vi "Test Method Execution Time recorded.vi"(8 "error in (no error)":errorcluster, 11 "Test Case In":refnum<class "Test Case Test.lvclass">) -> (0 "error out":errorcluster, 3 "Test Case Out":refnum<class "Test Case Test.lvclass">)   [LabVIEW 2020, in "Test Case Test.lvclass"]
uses:
  Test Case Test.lvclass
  C:/Program Files (x86)/National Instruments/LabVIEW 2020/vi.lib/Astemes/LUnit/Test Case.lvclass
  Test Doubles/Test Case Test Double/Methods.ctl
  source/Core/Result/Type.ctl
  <vilib>/Astemes/LUnit/Test Case.lvclass/Test Case.ctl
  <vilib>/Astemes/LUnit/Palette/Fail.vi
  <vilib>/Astemes/LUnit/Palette/Pass.vi
  <vilib>/Astemes/LUnit/Set Assertion Type.vi
  <vilib>/Astemes/LUnit/Add test result.vi
  <vilib>/Astemes/LUnit/LUnit Record Assertion Result.vi
  <vilib>/Astemes/LUnit/LUnit Aggregate Assertion Results.vi
  <vilib>/Astemes/LUnit/Method Result/LUnit Merge Status.vi
  <vilib>/Astemes/LUnit/LUnit Concatenate result strings.vi
  source/API/LUnit Test Case/LUnit Test Case.lvclass
  Test Doubles/Test Case Test Double/Test Case Test Double.lvclass
  <vilib>/Astemes/LUnit/Test Case.lvclass
  source/Core/Result/Result.lvlib
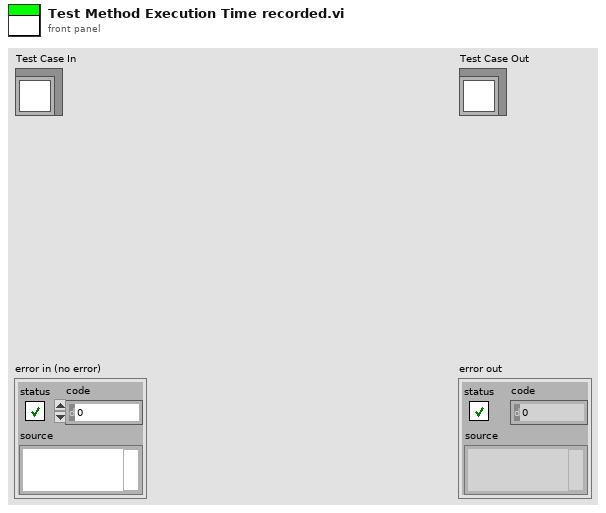
[diagram p1: front panel]
types:
  T1 = typedef "Test Case Test Double.lvclass/Methods.ctl" = enum16{"Test Failing Test.vi", "Test Passing Test.vi", "Test Error Test.vi", "Test Skip Test.vi", "Test Passing Pass If Test.vi", "Test Failing Pass If Test.vi", "Test Failing Fail If Test.vi", "Test Passing Fail If Test.vi", "Test Passing Pass If Error Test.vi", "Test Failing Pass If Error Test.vi", "Test Passing Fail If Error Test.vi", "Test Failing Fail If Error Test.vi", "Test Passing Pass If Equal Test.vi", "Test Failing Pass If Equal Test.vi", "Test Failing Fail If Equal Test.vi", "Test Passing Fail If Equal Test.vi", "Freezing Test.vi"}
  T2 = typedef "Result.lvlib/Result.ctl" = cluster{"Name":string, "Message":string, "Description":string, "Status":T3, "Result Type":T4, "Execution Time":dbl}
  T3 = typedef "Result.lvlib/Status.ctl" = enum16{"", "Passed", "Failed", "Error", "Skipped", "Setup Error", "Broken", "Teardown Error"}
  T4 = typedef "Result.lvlib/Type.ctl" = enum16{"Method", "Case", "Suite", "Pass", "Fail", "Skip", "Pass if", "Fail if", "Pass if Error", "Fail if Error", "Pass if Equal", "Fail if Equal"}
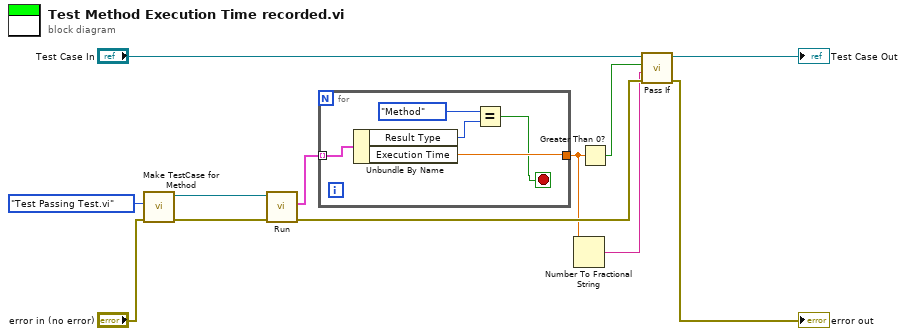
[diagram p0: block diagram]
diagram:
  n1 = call "Make TestCase for Method.vi"("error in (no error)"="error in (no error)", "Test Method"=Methods."Test Passing Test.vi") -> ("error out"=w8:errorcluster, "LUnit Test Case V2 out"=w9:refnum<class "LUnit Test Case.lvclass">)  [unwired: 8 in]
  n2 = call-dynamic "Run.vi"("error in (no error)"=w8, "LUnit Test Case In"=w9) -> ("error out"=w6:errorcluster, "Results"=w5:T2[])  [unwired: 6 in, 2 out]
  n3 = for {
    tunnel: w5 -> [w17] mode=indexing
    tunnel: [w16] -> w2
    stop <- w13 stop-if-true
    n4 = Unbundle By Name(w17) -> ("Result Type"=w14:T4, "Execution Time"=w16:dbl)
    n5 = Equal?(x=Type."Method" ("Result Type"), y=w14) -> (x = y?=w13:bool)
  }
  n6 = Number To Fractional String(number=w2) -> (F-format string=w1:string)  [unwired: 3 in]
  n7 = Greater Than 0?(x=w2) -> (x > 0?=w3:bool)
  n8 = call <vilib>:"Pass If.vi"("error in (no error)"=w6, "Message"=w1, "Pass?"=w3, "LUnit Test Case In"="Test Case In") -> ("error out"=→"error out":errorcluster, "LUnit Test Case Out"=→"Test Case Out":refnum<class "Test Case Test.lvclass">)  [unwired: 6 in]
